vi "TimeStamps.vi"(8 "Array 2":timestamp[](array[timestamp])=[timestamp(3381862363.917687 s since 1904-01-01), timestamp(3383140332.705 s since 1904-01-01), timestamp(3220380763.917687 s since 1904-01-01)], 9 "Array":T1(array[cluster])=[{"Time Stamp 2"=timestamp(3068992810 s since 1904-01-01), "Time Stamp"=timestamp(3383140282.158 s since 1904-01-01)}], 10 "Cluster":T2={"Time Stamp 2"=timestamp(3382380772.3951716 s since 1904-01-01), "Time Stamp"=timestamp(3382380763.917687 s since 1904-01-01)}, 11 "Time Stamp":timestamp=timestamp(3382639963.917687 s since 1904-01-01)) -> ()   [LabVIEW 2009]
panel:
  in  "stop":bool
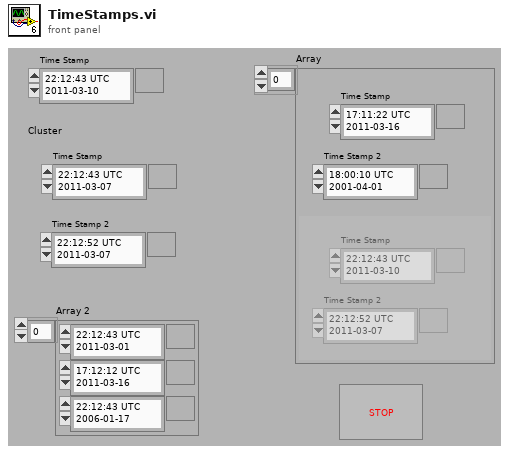
[diagram p1: front panel]
types:
  T1 = cluster{"Time Stamp 2":timestamp, "Time Stamp":timestamp}[]
  T2 = cluster{"Time Stamp 2":timestamp, "Time Stamp":timestamp}
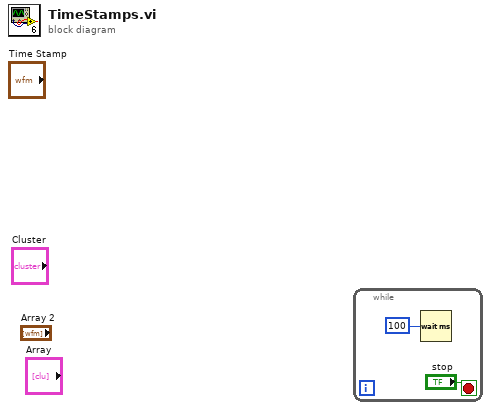
[diagram p0: block diagram]
diagram:
  n1 = while {
    stop <- "stop" stop-if-true
    n2 = Wait (ms)(milliseconds to wait=u32 100) -> ()  [unwired: 1 out]
  }
